vi "Configure.vi"(8 "error in (no error)":errorcluster, 11 "Cap Bank Server in":refnum<class "Cap Bank Server.lvclass">) -> (0 "error out":errorcluster, 3 "Cap Bank Server out":refnum<class "Cap Bank Server.lvclass">)   [LabVIEW 2015, in "Cap Bank Server.lvclass"]
uses:
  Cap Bank Server.lvclass
  Cap Bank Idot Measurement/Cap Bank Idot Measurement.lvclass
  Cap Bank Server.lvclass/Cap Bank Server.ctl
  <vilib>/ActorFramework/Actor/Actor.lvclass/Actor.ctl
  <vilib>/ActorFramework/Message Enqueuer/Message Enqueuer.lvclass/Message Enqueuer.ctl
  Mag Lab Measure Controller Messages/Log Status Update Msg/Log Status Update Msg.lvclass/Log Status Update Msg.ctl
  <vilib>/ActorFramework/Message Enqueuer/Init from Existing Queue.vi
  <vilib>/ActorFramework/Message Enqueuer/Enqueue.vi
  <vilib>/ActorFramework/Message Priority Queue/Priority Enqueue.vi
  Mag Lab Measure Controller.lvclass
  <vilib>/ActorFramework/Message Enqueuer/Message Enqueuer.lvclass
  Mag Lab Measure Controller Messages/Log Status Update Msg/Log Status Update Msg.lvclass
  <vilib>/ActorFramework/Actor/Actor.lvclass
  Mag Lab Measure Base/Mag Lab Measure Base.lvclass
  Cap Bank Interface/Cap Bank Interface.lvclass
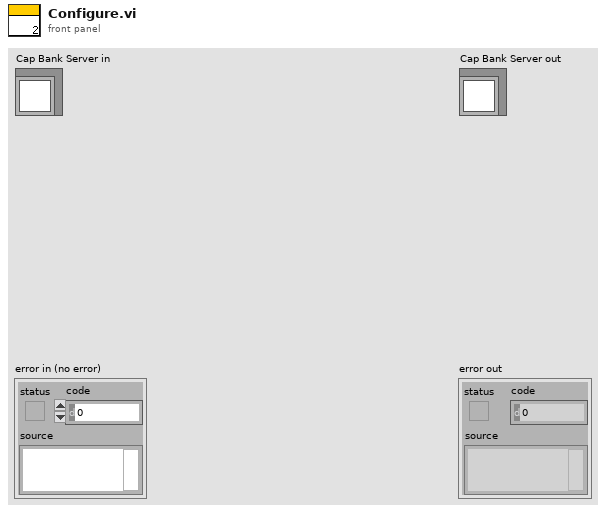
[diagram p1: front panel]
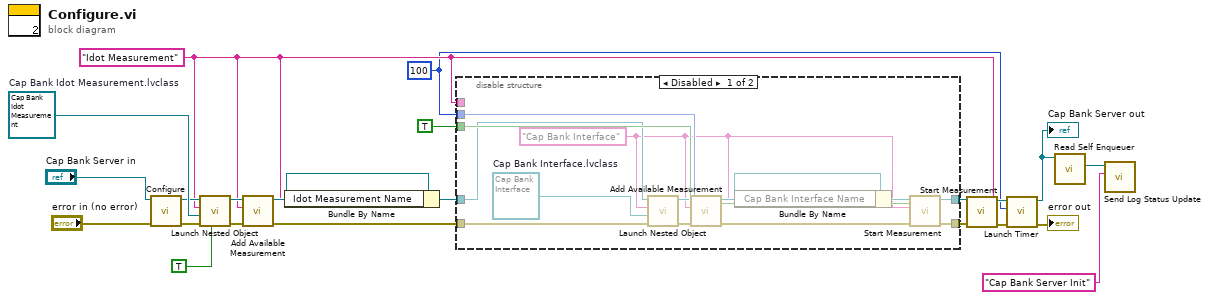
[diagram p0: block diagram]
diagram:
  w1 = u32 100 ("Poll delay")
  w6 = "Idot Measurement" ("Measurement name")
  w12 = refnum<class "Cap Bank Idot Measurement.lvclass"> refnum  # Cap Bank Idot Measurement.lvclass
  n1 = call-parent "Configure.vi"("error in (no error)"="error in (no error)", "Mag Lab Measure Controller in"="Cap Bank Server in") -> ("error out"=w15:errorcluster, "Mag Lab Measure Controller out"=w11:refnum<class "Cap Bank Server.lvclass">)  [unwired: 8 in]
  n2 = call "Launch Nested Object.vi"("Open Actor Core front panel? (F)"=TRUE, "error in (no error)"=w15, "Object"=w12, "name"=w6, "Mag Lab Measure Base in"=w11) -> ("error out"=w22:errorcluster, "Mag Lab Measure Base out"=w10:refnum<class "Cap Bank Server.lvclass">)  [unwired: 4 in, 1 out]
  n3 = call-dynamic "Add Available Measurement.vi"("error in (no error)"=w22, "Mag Lab Measurement"=w6, "Mag Lab Measure Controller in"=w10) -> ("error out"=w9:errorcluster, "Mag Lab Measure Controller out"=w8:refnum<class "Cap Bank Server.lvclass">)  [unwired: 7 in]
  n4 = Bundle By Name(cluster=w8, "Idot Measurement Name"=w6) -> (w7:refnum<class "Cap Bank Server.lvclass">)
  n5 = disable-structure shown="Disabled" {
    disable-tunnel: [w32 w36] -> w21
    disable-tunnel: [w31 w37] -> w20
    disable-tunnel: TRUE ("Acquire repeatedly") -> [w30 _]
    disable-tunnel: w1 -> [w29 _]
    disable-tunnel: w6 -> [_ _]
    disable-tunnel: w7 -> [w28 w36]
    disable-tunnel: w9 -> [w24 w37]
    frame Disabled {
      w26 = "Cap Bank Interface" ("Measurement name")
      w25 = refnum<class "Cap Bank Interface.lvclass"> refnum  # Cap Bank Interface.lvclass
      n6 = call "Launch Nested Object.vi"("error in (no error)"=w24, "Object"=w25, "name"=w26, "Mag Lab Measure Base in"=w28) -> ("error out"=w23:errorcluster, "Mag Lab Measure Base out"=w27:refnum<class "Cap Bank Server.lvclass">)  [unwired: 5 in, 1 out]
      n7 = call-dynamic "Add Available Measurement.vi"("error in (no error)"=w23, "Mag Lab Measurement"=w26, "Mag Lab Measure Controller in"=w27) -> ("error out"=w34:errorcluster, "Mag Lab Measure Controller out"=w35:refnum<class "Cap Bank Server.lvclass">)  [unwired: 7 in]
      n8 = Bundle By Name(cluster=w35, "Cap Bank Interface Name"=w26) -> (w33:refnum<class "Cap Bank Server.lvclass">)
      n9 = call-dynamic "Start Measurement.vi"(5:w29, 7:w30, "error in (no error)"=w34, "Measurement Name"=w26, "Mag Lab Measure Controller in"=w33) -> ("error out"=w31:errorcluster, "Mag Lab Measure Controller out"=w32:refnum<class "Cap Bank Server.lvclass">)  [unwired: 5 in]
    }
    frame Enabled {
    }
  }
  n10 = call-dynamic "Start Measurement.vi"("error in (no error)"=w20, "Measurement Name"=w6, "Mag Lab Measure Controller in"=w21) -> ("error out"=w3:errorcluster, "Mag Lab Measure Controller out"=w19:refnum<class "Cap Bank Server.lvclass">)  [unwired: 7 in]
  n11 = call-dynamic "Launch Timer.vi"("error in (no error)"=w3, "Timer period"=w1, "Mag Lab Measure Controller in"=w19) -> ("error out"=→"error out":errorcluster, "Mag Lab Measure Controller out"=w4:refnum<class "Cap Bank Server.lvclass">)  [unwired: 7 in]
  "Cap Bank Server out" <- w4
  n12 = call <vilib>:"Read Self Enqueuer.vi"("Actor"=w4) -> ("Self Enqueuer"=w18:refnum<class "Message Enqueuer.lvclass">)  [unwired: 10 in]
  n13 = call "Send Log Status Update.vi"("Status"="Cap Bank Server Init", "Message Enqueuer"=w18) -> ()  [unwired: 8 in, 2 out]
